vi "Write MonoID.vi"(8 "error in (no error)":errorcluster, 10 "MonoID":string, 11 "Monochromator in":refnum<class "Monochromator.lvclass">) -> (0 "error out":errorcluster, 3 "Monochromator out":refnum<class "Monochromator.lvclass">)   [LabVIEW 2016, in "Monochromator.lvclass"]
uses:
  Monochromator.lvclass
  Monochromator.lvclass/Monochromator.ctl
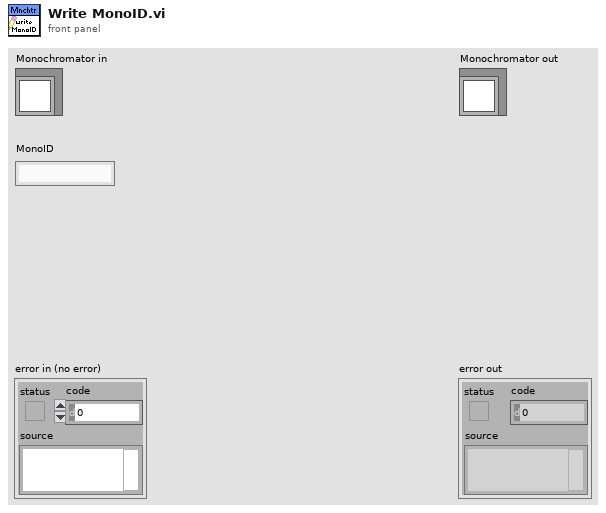
[diagram p1: front panel]
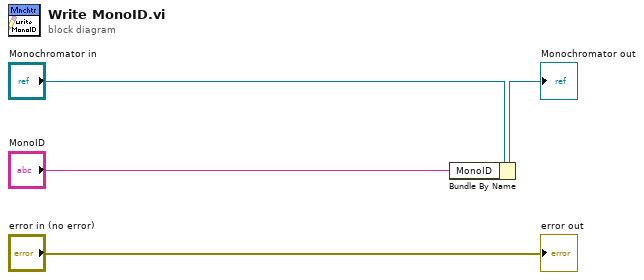
[diagram p0: block diagram]
diagram:
  n1 = Bundle By Name(cluster="Monochromator in", "MonoID"="MonoID") -> (→"Monochromator out":refnum<class "Monochromator.lvclass">)
  "error out" <- "error in (no error)"
